vi "FGV Get Key Value.vi"(7 "FGV Get INI Info":T1, 8 "error in (no error)":errorcluster, 9 "Key":string, 10 "Session":string, 11 "Ini File":T2(array[cluster])) -> (0 "error out":errorcluster, 1 "Number of Keys in Session":u32, 2 "All Keys and Values":cluster{"Key":string, "value":u32}[](array[cluster]), 3 "value":u32)   [LabVIEW 2021]
uses:
  FGV INI Values Action.ctl
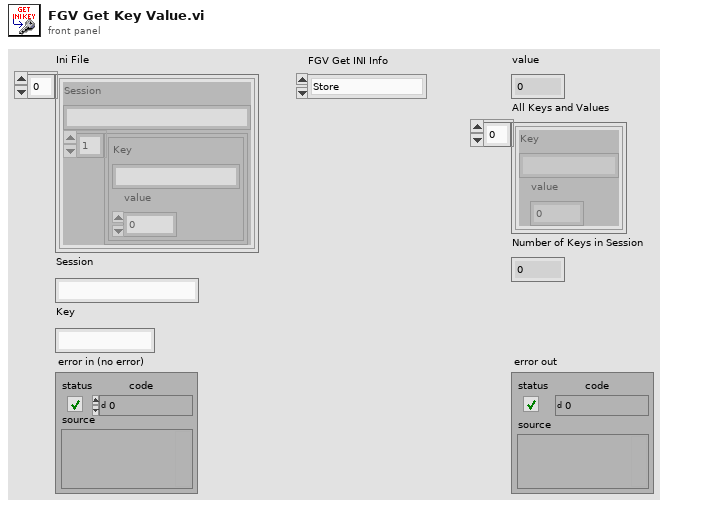
[diagram p1: front panel]
types:
  T1 = typedef "FGV INI Values Action.ctl" = enum16{"Store", "Get"}
  T2 = cluster{"Session":string, cluster{"Key":string, "value":u32}[]}[]
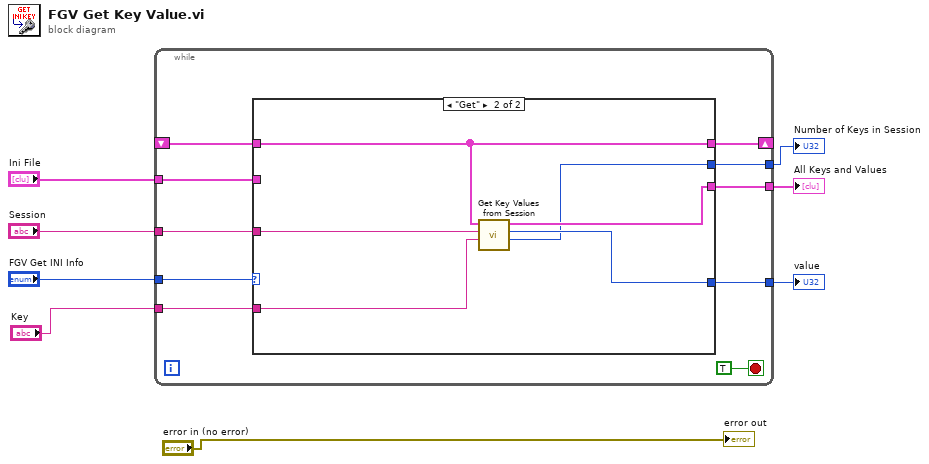
[diagram p0: block diagram]
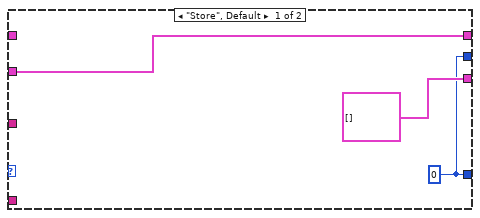
[diagram p2: hidden frame]
diagram:
  n1 = while {
    tunnel: "Ini File" -> [w17]
    tunnel: "FGV Get INI Info" -> [w18]
    shift-right: [w16] -> _
    shift-left: _ -> [w15]
    tunnel: "Session" -> [w14]
    tunnel: "Key" -> [w12]
    tunnel: [w11] -> w4
    tunnel: [w10] -> w3
    tunnel: [w9] -> w2
    stop <- TRUE stop-if-true
    n2 = case shown="\"Get\"" w18 {
      tunnel: w17 -> [w21 _]
      tunnel: [w21 w27] -> w16
      tunnel: w15 -> [_ w27]
      tunnel: w14 -> [_ w26]
      tunnel: w12 -> [_ w25]
      tunnel: [w19 w23] -> w11
      tunnel: [cluster{"Key":string, "value":u32}[] [] w24] -> w10
      tunnel: [w19 w22] -> w9
      frame "Store", Default {
        w19 = u32 0 ("value")
      }
      frame "Get" {
        n3 = call "Get Key Values from Session.vi"("Key"=w25, "Session"=w26, "Ini File"=w27) -> ("Number of Keys"=w22:i32, "Search Key Value"=w23:u32, "Keys Values in Session"=w24:cluster{"Key":string, "value":u32}[])  [unwired: 6 in]
      }
    }
  }
  "value" <- w4
  "All Keys and Values" <- w3
  "Number of Keys in Session" <- w2
  "error out" <- "error in (no error)"
